vi "1D DBL Array Binary.vi"(4 "Option 2":i64=2, 6 "Option 1":i64, 10 "Path In":path) -> (2 "Data Out":dbl[](array[numeric]) format="%#_f")   [LabVIEW 2022 SP3]
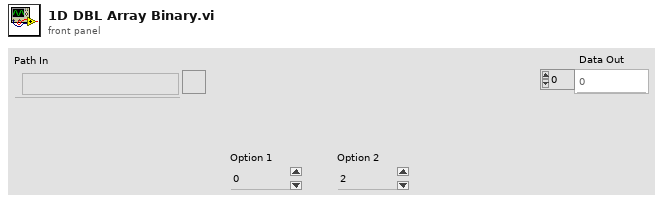
[diagram p1: front panel]
types:
  T1 = enum16{"big-endian, network order", "native, host order", "little-endian"}
  T2 = enum16{"open", "replace", "create", "open or create", "replace or create", "replace or create with confirmation"}
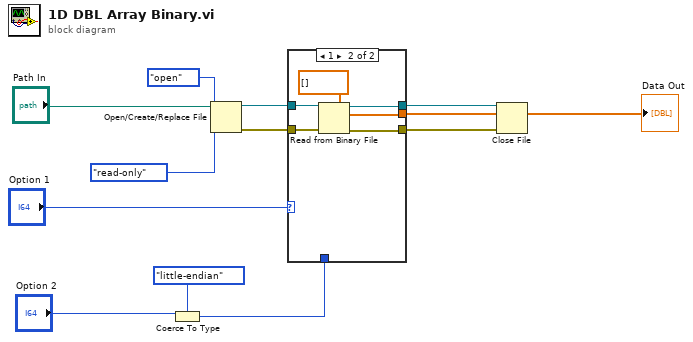
[diagram p0: block diagram]
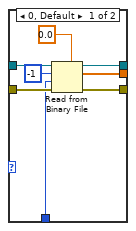
[diagram p2: hidden frame]
diagram:
  n1 = Coerce To Type(0:"Option 2", 1:T1."little-endian" ("byte order (0:big-endian, network order)")) -> (2:w1:T1)
  n2 = Open/Create/Replace File(file path (use dialog)="Path In", operation (0:open)=T2."open", access (0:read/write)=enum16{"read/write", "read-only", "write-only"}."read-only") -> (refnum out=w10:refnum<file>, error out=w9:errorcluster)  [unwired: 3 in, 1 out]
  n3 = case shown="1" "Option 1" {
    tunnel: w10 -> [w20 w26]
    tunnel: w9 -> [w19 w24]
    tunnel: w1 -> [w18 _]
    tunnel: [w15 w25] -> w8
    tunnel: [w14 w23] -> w7
    tunnel: [w13 w21] -> w5
    frame 0, Default {
      n4 = Read from Binary File(5:0.0, 8:w19, 9:w18, 10:-1 ("count (1)"), 11:w20) -> (0:w14:errorcluster, 2:w13:dbl[], 3:w15:refnum<file>)  [unwired: 1 in, 1 out]
    }
    frame 1 {
      n5 = Read from Binary File(5:dbl[] [], 8:w24, 11:w26) -> (0:w23:errorcluster, 2:w21:dbl[], 3:w25:refnum<file>)  [unwired: 3 in, 1 out]
    }
  }
  "Data Out" <- w5
  n6 = Close File(refnum=w8, error in=w7) -> ()  [unwired: 2 out]
